vi "Add While Loop.vi"(8 "error in (no error)":errorcluster, 9 "Section":enum16{"Main", "Setup", "Cleanup"}(ring), 10 "Condition":string, 11 "RT Sequence Ref in":refnum<k24>) -> (0 "error out":errorcluster, 2 "While Loop Ref":refnum<k24>, 3 "RT Sequence Ref out":refnum<k24>)   [LabVIEW 2016, in "RT Sequence Creator API.lvlib"]
uses:
  RT Sequence Creator API.lvlib
  NationalInstruments.VeriStand.RealTimeSequenceDefinitionApi
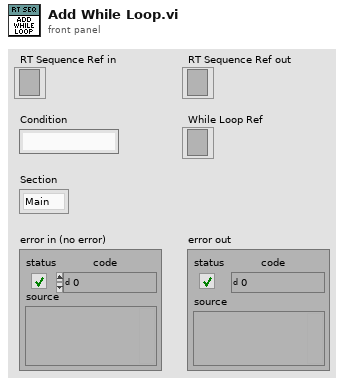
[diagram p1: front panel]
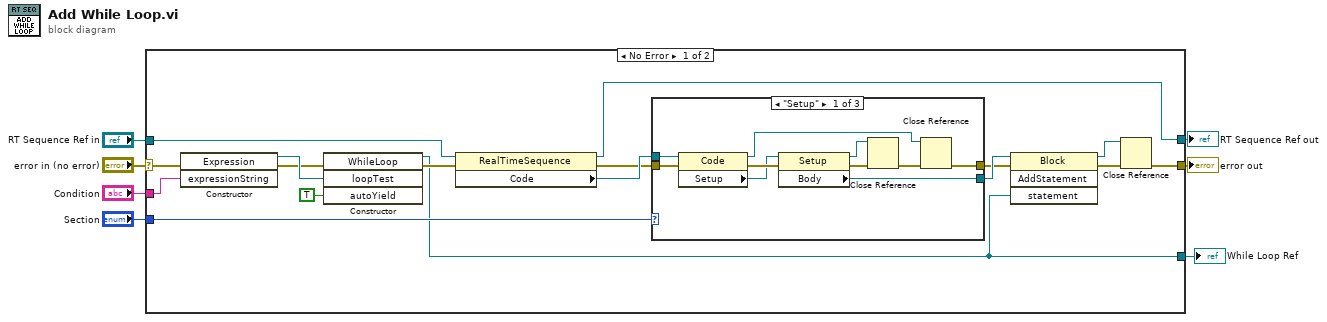
[diagram p0: block diagram]
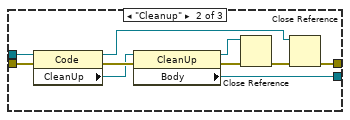
[diagram p2: hidden frame]
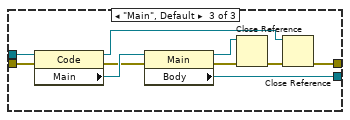
[diagram p3: hidden frame]
diagram:
  n1 = case shown="No Error" "error in (no error)" {
    selector: "error in (no error)" -> [w18 w55]
    tunnel: "RT Sequence Ref in" -> [w24 w56]
    tunnel: [w9 w55] -> w5
    tunnel: [w20 w56] -> w4
    tunnel: "Section" -> [w21 _]
    tunnel: "Condition" -> [w16 _]
    tunnel: [w11 _] -> w1
    frame No Error {
      n2 = constructor class="Expression"(error in=w18, "expressionString"=w16) -> (reference out=w17:refnum<k24>, error out=w15:errorcluster)  [unwired: 2 in, 2 out]
      n3 = constructor class="WhileLoop"(error in=w15, "loopTest"=w17, "autoYield"=TRUE) -> (reference out=w11:refnum<k24>, error out=w19:errorcluster)  [unwired: 2 in, 3 out]
      n4 = property class="RealTimeSequence"(reference=w24, error in=w19) -> (reference out=w20:refnum<k24>, error out=w22:errorcluster, "Code"=w23:refnum<k24>)
      n5 = case shown="\"Setup\"" w21 {
        tunnel: w23 -> [w34 w44 w54]
        tunnel: w22 -> [w33 w43 w53]
        tunnel: [w32 w41 w46] -> w12
        tunnel: [w30 w35 w45] -> w13
        frame "Setup" {
          n6 = property class="Code"(reference=w34, error in=w33) -> (reference out=w31:refnum<k24>, error out=w29:errorcluster, "Setup"=w28:refnum<k24>)
          n7 = property class="Setup"(reference=w28, error in=w29) -> (reference out=w25:refnum<k24>, error out=w27:errorcluster, "Body"=w30:refnum<k24>)
          n8 = Close Reference(reference=w25, error in (no error)=w27) -> (error out=w26:errorcluster)
          n9 = Close Reference(reference=w31, error in (no error)=w26) -> (error out=w32:errorcluster)
        }
        frame "Cleanup" {
          n10 = property class="Code"(reference=w44, error in=w43) -> (reference out=w40:refnum<k24>, error out=w39:errorcluster, "CleanUp"=w38:refnum<k24>)
          n11 = property class="CleanUp"(reference=w38, error in=w39) -> (reference out=w37:refnum<k24>, error out=w36:errorcluster, "Body"=w35:refnum<k24>)
          n12 = Close Reference(reference=w37, error in (no error)=w36) -> (error out=w42:errorcluster)
          n13 = Close Reference(reference=w40, error in (no error)=w42) -> (error out=w41:errorcluster)
        }
        frame "Main", Default {
          n14 = property class="Code"(reference=w54, error in=w53) -> (reference out=w47:refnum<k24>, error out=w51:errorcluster, "Main"=w52:refnum<k24>)
          n15 = property class="Main"(reference=w52, error in=w51) -> (reference out=w48:refnum<k24>, error out=w50:errorcluster, "Body"=w45:refnum<k24>)
          n16 = Close Reference(reference=w48, error in (no error)=w50) -> (error out=w49:errorcluster)
          n17 = Close Reference(reference=w47, error in (no error)=w49) -> (error out=w46:errorcluster)
        }
      }
      n18 = invoke class="Block" method="AddStatement"(reference=w13, error in=w12, "statement"=w11) -> (reference out=w8:refnum<k24>, error out=w10:errorcluster)  [unwired: 1 in, 2 out]
      n19 = Close Reference(reference=w8, error in (no error)=w10) -> (error out=w9:errorcluster)
    }
    frame Error {
    }
  }
  "RT Sequence Ref out" <- w4
  "error out" <- w5
  "While Loop Ref" <- w1
